vi "Stop Polling.vi"(8 "Error In":errorcluster, 11 "CS++BaseActor in":refnum<class "CS++BaseActor.lvclass">) -> (0 "Error Out":errorcluster, 3 "CS++BaseActor out":refnum<class "CS++BaseActor.lvclass">)   [LabVIEW 2015, in "CS++BaseActor.lvlib" / "CS++BaseActor.lvclass"]
doc: "Set attribute <b>Polling Fast</b> to false."
uses:
  CS++BaseActor.lvclass
  Classes/CS++ProcessVariables/ProcessVariable/PV.lvclass
  CS++BaseActor.lvclass/CS++BaseActor.ctl
  <vilib>/ActorFramework/Time-Delayed Send Message/Time-Delay Override Options.ctl
  Classes/CS++ProcessVariables/ProcessVariable/PV.lvclass/PV.ctl
  Classes/CS++ProcessVariables/ProcessVariable/Write Timestamp.vi
  Classes/CS++ProcessVariables/ProcessVariable/Write Data.vi
  Classes/CS++ProcessVariables/PVConnection/PVConnection.lvclass
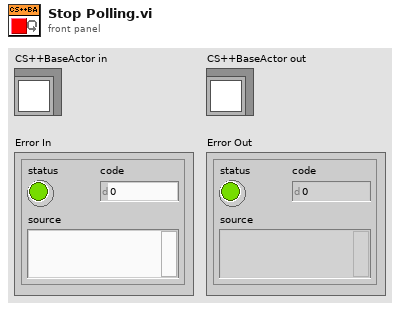
[diagram p1: front panel]
types:
  T1 = typedef "Time-Delay Override Options.ctl" = enum16{"Send next copy now", "Skip next scheduled copy", "Send next copy now and stop all further copies", "Stop all further copies"}
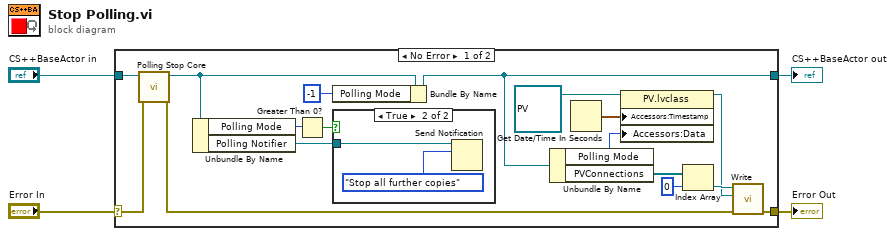
[diagram p0: block diagram]
diagram:
  n1 = case shown="No Error" "Error In" {
    selector: "Error In" -> [w6 w25]
    tunnel: [w9 w25] -> w3
    tunnel: [w10 w24] -> w1
    tunnel: "CS++BaseActor in" -> [w8 w24]
    frame No Error {
      n2 = call-dynamic "Polling Stop Core.vi"("Error In"=w6, "CS++BaseActor in"=w8) -> ("Error Out"=w5:errorcluster, "CS++BaseActor out"=w7:refnum<class "CS++BaseActor.lvclass">)  [unwired: 8 in]
      n3 = Unbundle By Name(w7) -> ("Polling Mode"=w20:i32, "Polling Notifier"=w18:refnum<notifier>)
      n4 = Greater Than 0?(x=w20) -> (x > 0?=w19:bool)
      n5 = Bundle By Name(cluster=w7, "Polling Mode"=-1) -> (w10:refnum<class "CS++BaseActor.lvclass">)
      n6 = case shown="True" w19 {
        tunnel: w18 -> [_ w23]
        frame False {
        }
        frame True {
          n7 = Send Notification(notification=Time-Delay_Override_Options."Stop all further copies", notifier=w23) -> ()  [unwired: 1 in, 2 out]
        }
      }
      n8 = Unbundle By Name(w10) -> ("Polling Mode"=w13:i32, "PVConnections"=w16:refnum<class "PVConnection.lvclass">[])
      n9 = Get Date/Time In Seconds() -> (seconds since 1Jan1904=w14:timestamp)
      n10 = property class="PV.lvclass"(reference=refnum<class "PV.lvclass"> refnum ("CS++ProcessVariables.lvlib:PV.lvclass"), "Accessors:Timestamp"=w14, "Accessors:Data"=w13) -> (reference out=w11:refnum<class "PV.lvclass">)  [unwired: 1 in, 1 out]
      n11 = Index Array(array=w16, index=0) -> (element=w12:refnum<class "PVConnection.lvclass">)
      n12 = call "Write.vi"("error in (no error)"=w5, "PV"=w11, "PVConnection in"=w12) -> ("error out"=w9:errorcluster)  [unwired: 7 in, 1 out]
    }
    frame Error {
    }
  }
  "Error Out" <- w3
  "CS++BaseActor out" <- w1
